vi "About Dialog.vi"(2 "AppVer":string="SW Rev. SFTS_1.0/13-0902-0", 3 "Main UI Ref":refnum<vi>) -> ()   [LabVIEW 2019]
doc: "Developed by Kevin Thompson\nThompson Engineering, LLC\nkevin@thompsonengineering.net"
panel:
  in  "OK":bool
  # "IHS\nInverter Health Scanner"
  # "Produced for inifiniRel Corporation\nIHS Software Application, Copyright 2020\nAll Rights Reserved\n\n\nAll Software Design and Development\nby Kevin Thompson\nThompson Engineering, LLC"
  # "Portions of this software developed and provided by\nthe following organizations, with All Rights Reserved."
  # "National Instruments, Inc.\nThompson Engineering, LLC\nOpen Source LabVIEW Software Movement\nMoore Good Ideas, Inc."
  # "CLICK HERE"
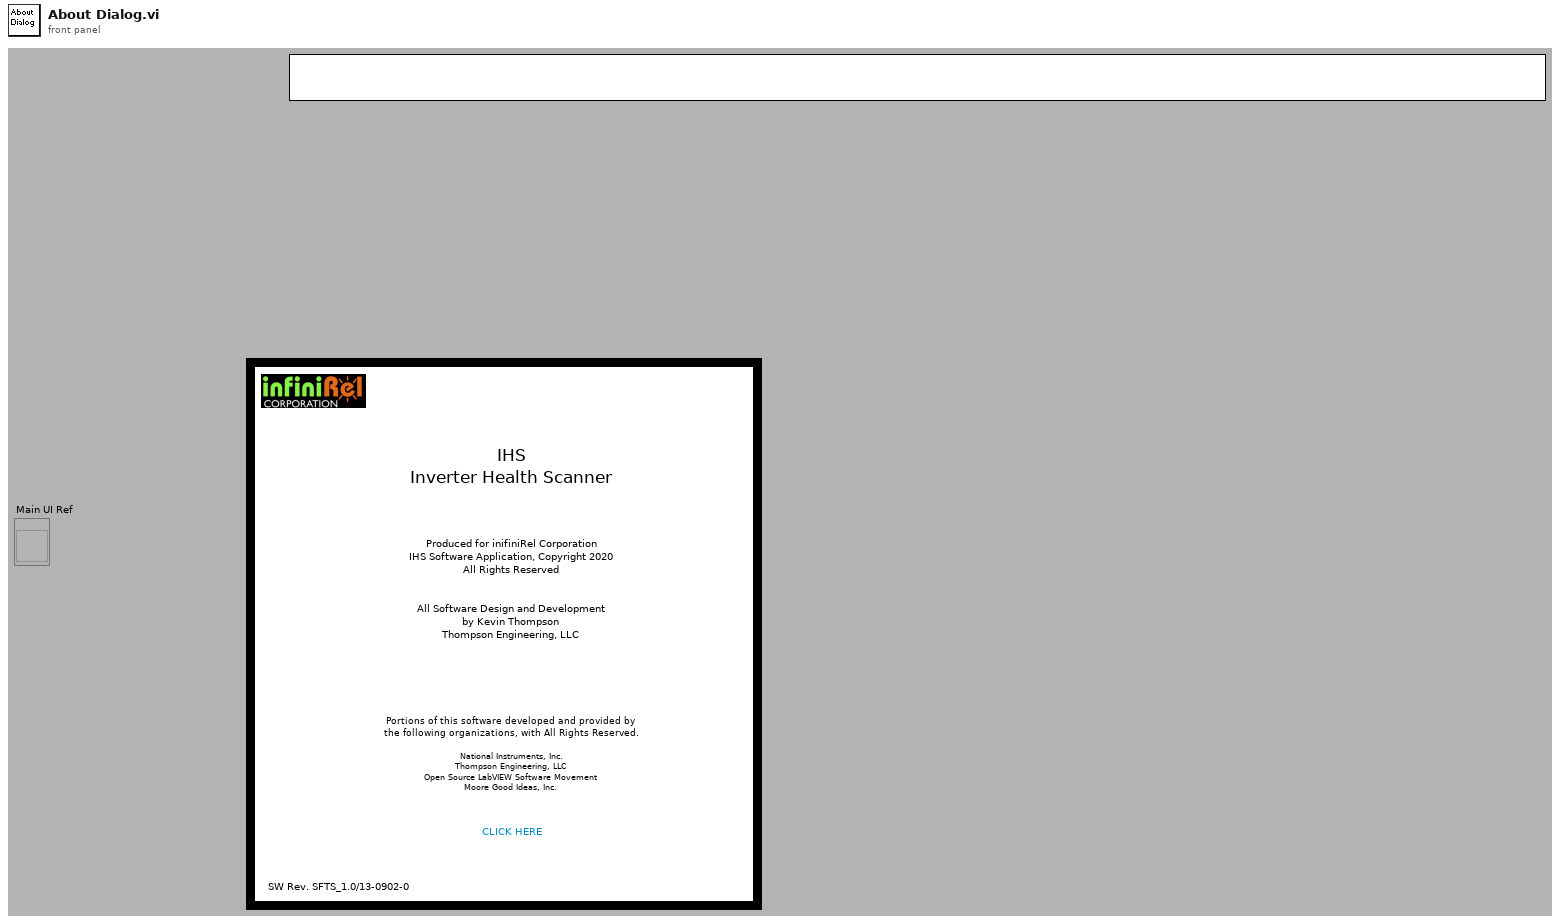
[diagram p1: front panel]
types:
  T1 = enum32{"Invalid", "Default", "Floating", "Floating/Auto-Hide", "Modal"}
  T2 = enum32{"Invalid", "Standard", "Closed", "Hidden", "Minimized", "Maximized"}
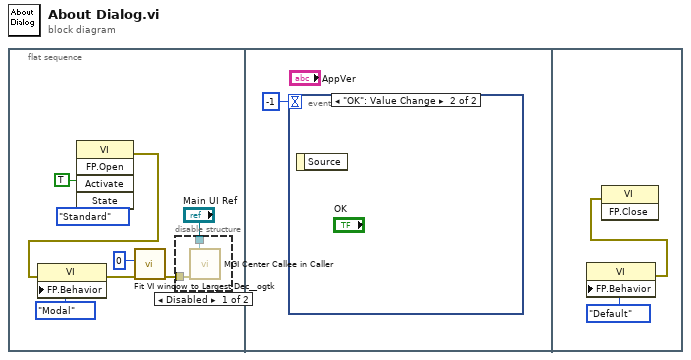
[diagram p0: block diagram]
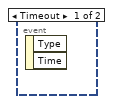
[diagram p3: hidden frame]
diagram:
  n1 = flat-sequence {
    frame #0 {
      n2 = invoke class="VI" method="FP.Open"("Activate"=TRUE ("Activate?"), "State"=T2."Standard") -> (error out=w5:errorcluster)  [unwired: 3 in, 4 out]
      n3 = property class="VI"(error in=w5, "FP.Behavior"=T1."Modal" ("Front Panel Window:Behavior")) -> (error out=w4:errorcluster)  [unwired: 1 in, 1 out]
      n4 = call <userlib>:"Fit VI window to Largest Dec__ogtk.vi"("error in (no error)"=w4, "border spacing (2 px)"=0) -> ("error out"=w2:errorcluster)  [unwired: 4 in, 1 out]
      n5 = disable-structure shown="Disabled" {
        disable-tunnel: w2 -> [w10 _]
        disable-tunnel: "Main UI Ref" -> [w9 _]
        frame Disabled {
          n6 = call <userlib>:"MGI Center Callee in Caller.vi"("Error In"=w10, "Caller VI Refnum (Callee's Caller)"=w9) -> ()  [unwired: 9 in, 1 out]
        }
        frame Enabled {
        }
      }
    }
    frame #1 {
      n7 = event shown="[1] \"OK\": Value Change" {
        selector: _ -> [_ _]
        dyn-events: _ -> [_ _]
        timeout: -1 -> [_ _]
        event Timeout {
          n8 = event-data() -> ()  [unwired: 1 in, 2 out]
        }
        event "OK": Value Change {
          n9 = event-data() -> ()  [unwired: 1 in, 1 out]
        }
      }
    }
    frame #2 {
      n10 = property class="VI"("FP.Behavior"=T1."Default" ("Front Panel Window:Behavior")) -> (error out=w12:errorcluster)  [unwired: 2 in, 1 out]
      n11 = invoke class="VI" method="FP.Close"(error in=w12) -> ()  [unwired: 2 in, 3 out]
    }
  }
